vi "RPM Simulator.vi"(8 "error in (no error)":errorcluster, 11 "Acquisition Mertrics in":T1) -> (0 "error out":errorcluster, 3 "Acquisition Mertrics out":T1)   [LabVIEW 2026, in "Acquisition.lvlib"]
uses:
  Acquisition.lvlib
  Controls/Acquisition Metrics.ctl
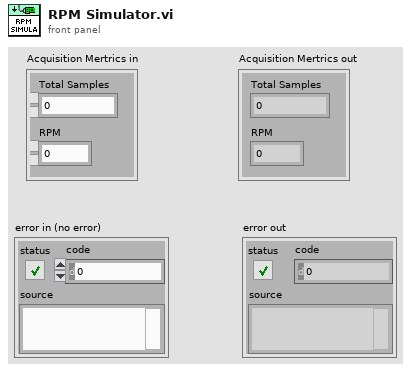
[diagram p1: front panel]
types:
  T1 = typedef "Acquisition.lvlib/Acquisition Metrics.ctl" = cluster{"Total_Samples":i64, "RPM":dbl}
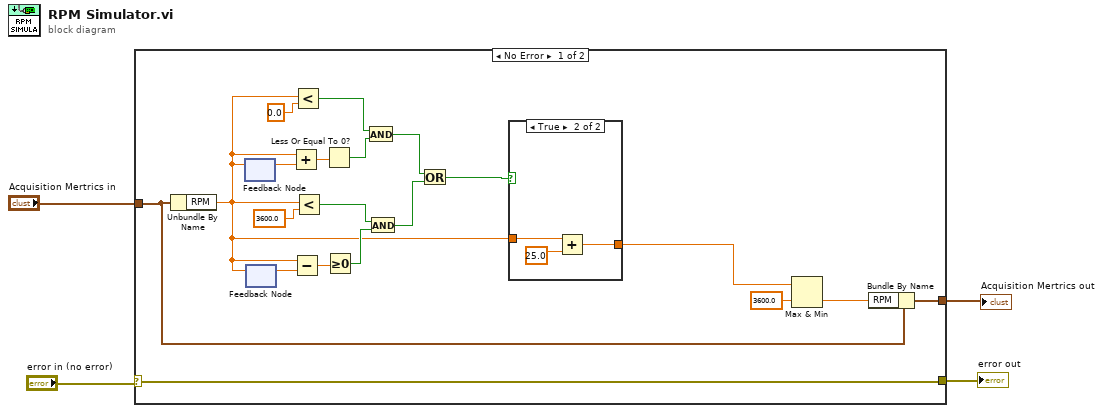
[diagram p0: block diagram]
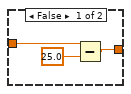
[diagram p2: hidden frame]
diagram:
  n1 = case shown="No Error" "error in (no error)" {
    selector: "error in (no error)" -> [w21 w31]
    tunnel: "Acquisition Mertrics in" -> [w18 w32]
    tunnel: [w22 w32] -> w3
    tunnel: [w21 w31] -> w1
    frame No Error {
      n2 = Unbundle By Name(w18) -> ("RPM"=w8:dbl)
      n3 = feedback #1() -> (w10:dbl)  [unwired: 1 in]
      n4 = feedback-in #1(w8) -> ()
      n5 = feedback-in #2(w8) -> ()
      n6 = feedback #2() -> (w15:dbl)  [unwired: 1 in]
      n7 = Add(x=w8, y=w10) -> (x+y=w12:dbl)
      n8 = Subtract(x=w8, y=w15) -> (x-y=w17:dbl)
      n9 = Less?(x=w8, y=0.0) -> (x < y?=w9:bool)
      n10 = Less?(x=w8, y=3600.0) -> (x < y?=w14:bool)
      n11 = Less Or Equal To 0?(x=w12) -> (x <= 0?=w11:bool)
      n12 = Greater Or Equal To 0?(x=w17) -> (x >= 0?=w16:bool)
      n13 = And(x=w9, y=w11) -> (x .and. y?=w7:bool)
      n14 = And(x=w14, y=w16) -> (x .and. y?=w6:bool)
      n15 = Or(x=w7, y=w6) -> (x .or. y?=w5:bool)
      n16 = case shown="True" w5 {
        tunnel: w8 -> [w27 w28]
        tunnel: [w25 w29] -> w19
        frame False {
          n17 = Subtract(x=w27, y=25.0) -> (x-y=w25:dbl)
        }
        frame True {
          n18 = Add(x=w28, y=25.0 ("x")) -> (x+y=w29:dbl)
        }
      }
      n19 = Max & Min(x=w19, y=3600.0) -> (min(x,y)=w24:dbl)  [unwired: 1 out]
      n20 = Bundle By Name(cluster=w18, "RPM"=w24) -> (w22:T1)
    }
    frame Error {
    }
  }
  "Acquisition Mertrics out" <- w3
  "error out" <- w1
